vi "UploadSource.vi"(8 "error in (no error)":errorcluster, 11 "Vision in":refnum<class "Vision.lvclass">) -> (0 "error out":errorcluster, 3 "Vision out":refnum<class "Vision.lvclass">)   [LabVIEW 2021, in "Vision.lvlib" / "Vision.lvclass"]
uses:
  Vision.lvclass
  C:/Program Files (x86)/National Instruments/LabVIEW 2021/vi.lib/ActorFramework/Actor/Actor.lvclass
  <vilib>/ActorFramework/Actor/Actor.lvclass/Actor.ctl
  Vision.lvclass/Vision.ctl
  Vision Messages/CapturedImage Msg/CapturedImage Msg.lvclass/CapturedImage Msg.ctl
  <vilib>/ActorFramework/Message Enqueuer/Message Enqueuer.lvclass/Message Enqueuer.ctl
  <vilib>/ActorFramework/Message Enqueuer/Enqueue.vi
  Vision Messages/CapturedImage Msg/CapturedImage Msg.lvclass
  C:/Program Files (x86)/National Instruments/LabVIEW 2021/vi.lib/ActorFramework/Message/Message.lvclass
  <vilib>/ActorFramework/Message Priority Queue/Priority Enqueue.vi
  <vilib>/ActorFramework/Message Enqueuer/Message Enqueuer.lvclass
  <vilib>/ActorFramework/Actor/Actor.lvclass
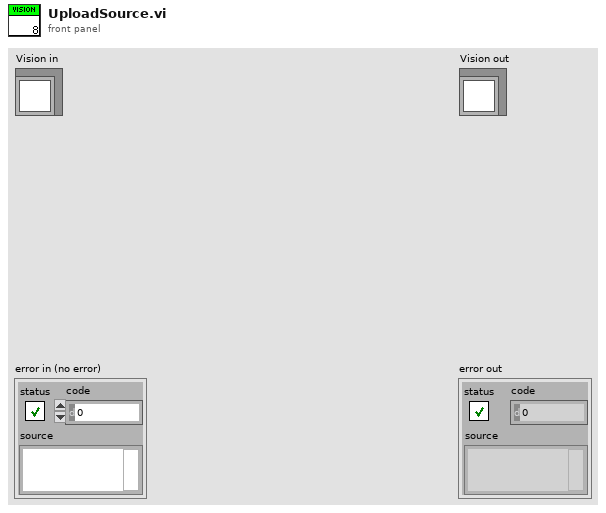
[diagram p1: front panel]
types:
  T1 = cluster{"guid":string, "images":cluster{"source":string, "rois":string[]}}
  T2 = typedef "IMAQ Image.ctl" = refnum<image>
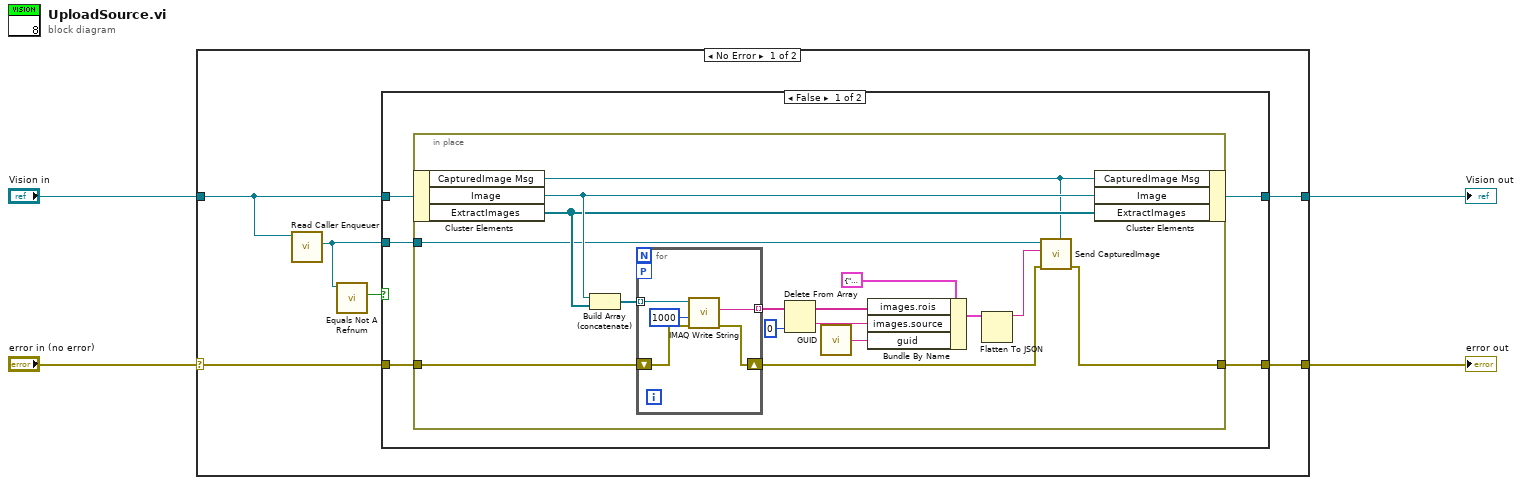
[diagram p0: block diagram]
diagram:
  n1 = case shown="No Error" "error in (no error)" {
    selector: "error in (no error)" -> [w8 w40]
    tunnel: [w7 w40] -> w1
    tunnel: [w9 w39] -> w2
    tunnel: "Vision in" -> [w10 w39]
    frame No Error {
      n2 = call <vilib>:"Read Caller Enqueuer.vi"("Actor"=w10) -> ("Caller Enqueuer"=w5:refnum<class "Message Enqueuer.lvclass">)  [unwired: 10 in]
      n3 = call <vilib>:"Equals Not A Refnum.vi"("Message Enqueuer"=w5) -> ("Not a refnum?"=w6:bool)  [unwired: 10 in]
      n4 = case shown="False" w6 {
        tunnel: w10 -> [w15 w38]
        tunnel: [w14 w38] -> w9
        tunnel: w8 -> [w13 w37]
        tunnel: [w11 w37] -> w7
        tunnel: w5 -> [w12 _]
        frame False {
          n5 = in-place {
            in-place-border: w13 -> [w28]
            in-place-border: w12 -> [w20]
            in-place-border: [w18] -> w11
            n6 = in-place-cluster #1(w15) -> ("CapturedImage Msg"=w26:refnum<class "CapturedImage Msg.lvclass">, "Image"=w31:T2, "ExtractImages"=w30:T2[])
            n7 = Build Array (concatenate)(w31, w30) -> (w29:T2[])
            n8 = for {
              tunnel: w29 -> [w36] mode=indexing
              shift-right: [w34] -> w19
              shift-left: w28 -> [w35]
              tunnel: [w33] -> w27 mode=indexing
              workers-P: _ -> [_]
              n9 = call-poly "IMAQ Write String"("error in (no error)"=w35, "Image Quality"=u32 1000, "Image"=w36) -> ("error out"=w34:errorcluster, "FileString"=w33:string)  [unwired: 6 in, 1 out]
            }
            n10 = Delete From Array(array=w27, index=0) -> (deleted portion=w24:string, array with subset deleted=w23:string[])  [unwired: 1 in]
            n11 = call "GUID.vi"() -> ("Guid"=w16:string)  [unwired: 1 in]
            n12 = Bundle By Name(cluster=T1 {"guid"="", "images"={"source"="", "rois"=[]}}, "images.rois"=w23, "images.source"=w24, "guid"=w16) -> (w22:T1)
            n13 = Flatten To JSON(anything=w22) -> (JSON string=w21:string)  [unwired: 2 in, 1 out]
            n14 = call "Send CapturedImage.vi"("Message Type"=w26, "error in (no error)"=w19, "JSON"=w21, "Message Enqueuer"=w20) -> ("error out"=w18:errorcluster)  [unwired: 6 in, 1 out]
            n15 = in-place-cluster #1("CapturedImage Msg"=w26, "Image"=w31, "ExtractImages"=w30) -> (w14:refnum<class "Vision.lvclass">)
          }
        }
        frame True {
        }
      }
    }
    frame Error {
    }
  }
  "error out" <- w1
  "Vision out" <- w2
